vi "RT_Network Write Loop.vi"(8 "error in":errorcluster, 11 "Main Data":T1) -> (0 "error out":errorcluster)   [LabVIEW 2018]
uses:
  Data Def/RT_Main Data.ctl
  Data Def/RT_FPGA VI Reference.ctl
  Data Def/RT_Request Data.ctl
  Com/WebSockets/Data Def/Websocket Command.ctl
panel:
  out "x-y":u32
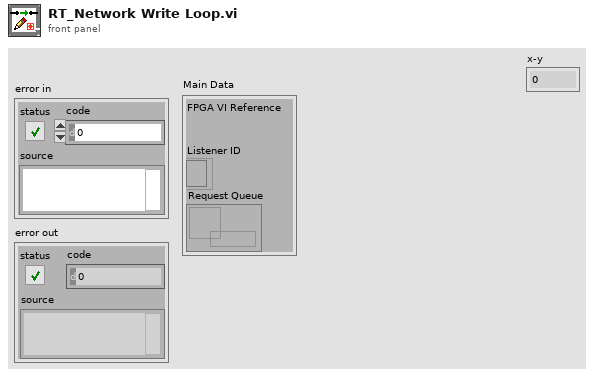
[diagram p1: front panel]
types:
  T1 = typedef "RT_Main Data.ctl" = cluster{"FPGA VI Reference":T2, "Listener ID":refnum<k5>, "Request Queue":refnum<queue>}
  T2 = typedef "RT_FPGA VI Reference.ctl" = refnum<k20>
  T3 = typedef "Websocket Command.ctl" = cluster{"Command":string, "Data":string}
  T4 = typedef "RT_Request Data.ctl" = cluster{"Connection ID":refnum<k5>, "Command":string, "Data":string}
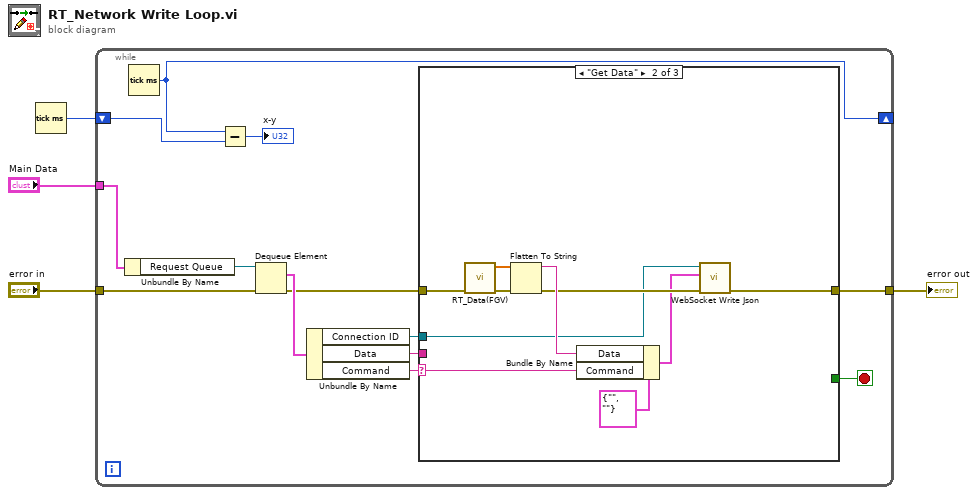
[diagram p0: block diagram]
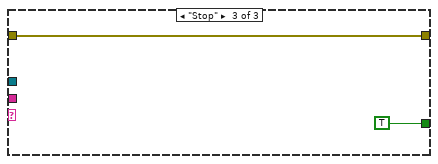
[diagram p3: hidden frame]
diagram:
  n1 = Tick Count (ms)() -> (millisecond timer value=w1:u32)
  n2 = while {
    tunnel: "Main Data" -> [w17]
    tunnel: "error in" -> [w15]
    tunnel: [w9] -> w2
    shift-right: [w7] -> _
    shift-left: w1 -> [w6]
    stop <- w8 stop-if-true
    n3 = Unbundle By Name(w17) -> ("Request Queue"=w16:refnum<queue>)
    n4 = Tick Count (ms)() -> (millisecond timer value=w7:u32)
    n5 = Subtract(x=w7, y=w6) -> (x-y=→"x-y":u32)
    n6 = Dequeue Element(queue=w16, error in (no error)=w15) -> (element=w14:T4, error out=w10:errorcluster)  [unwired: 1 in, 2 out]
    n7 = Unbundle By Name(w14) -> ("Connection ID"=w11:refnum<k5>, "Data"=w12:string, "Command"=w13:string)
    n8 = case shown="\"Get Data\"" w13 {
      selector: w13 -> [_ w24 _]
      tunnel: w12 -> [_ _ _]
      tunnel: w11 -> [_ w20 _]
      tunnel: w10 -> [w18 w28 w30]
      tunnel: [w18 w19 w30] -> w9
      tunnel: [_ _ TRUE] -> w8
      frame Default {
      }
      frame "Get Data" {
        n9 = call "RT_Data(FGV).vi"("error in"=w28) -> ("error out"=w27:errorcluster, "Data Out"=w26:dbl[])  [unwired: 9 in]
        n10 = Flatten To String(anything=w26, error in (no error)=w27) -> (data string=w23:string, error out=w22:errorcluster)  [unwired: 2 in, 1 out]
        n11 = Bundle By Name(cluster=T3 {"Command"="", "Data"=""} ("Websocket Command"), "Data"=w23, "Command"=w24) -> (w21:T3)
        n12 = call "WebSocket Write Json.vi"("error in"=w22, "Websocket Command"=w21, "WebSocket Connection in"=w20) -> ("error out"=w19:errorcluster)  [unwired: 7 in, 1 out]
      }
      frame "Stop" {
      }
    }
  }
  "error out" <- w2
